vi "InternalGenerateValObjXML.vi"(6 "static class name":string, 7 "Class version":T1, 10 "Parent After Child":string, 11 "Parent Before Child":string) -> (0 "After Child":string, 1 "Object as XML":string, 3 "Before Child":string)   [LabVIEW 2015, in "OpenG_Value_Object.lvclass"]
doc: "A method used internally by the class to construct XML."
uses:
  <userlib>/_OpenG.lib/openg_object/openg_value_object.llb/OpenG_Value_Object.lvclass
  <userlib>/_OpenG.lib/openg_object/openg_object.llb/OpenG_Object.lvclass
panel:
  # "Please visit http://www.OpenG.org to learn about the\nOpen Source LabVIEW software movement.\n\nNOTICE -- YOU MUST LEAVE THIS NOTICE IN PLACE.  PER THE TERMS OF THE LICENSE BELOW, YOU MAY SUBLICENSE THIS SOFTWARE \nIN ANY WAY THAT DOES NOT CONFLICT WITH THIS LICENSE.\n\n### BSD License (http://www.opensource.org/licenses/bsd-license.php) Begin ###\n\nCopyright (c) 2007, Tomi Maila\nCopyright (c) 2007, Endevo AB\n\n\nAll rights reserved.\n\nRedistribution and use in source and binary forms, with or without modification, are permitted provided that the following conditions are met:\n\n    * Redistributions of source code must retain the above copyright notice, this list of conditions and the following disclaimer.\n    * Redistributions in binary form must reproduce the above copyright notice, this list of conditions and the following disclaimer in the \n       documentation and/or other materials provided with the distribution.\n    * Neither the name of Endevo AB nor the names of the contributors may be used to endorse or promote products derived\n       from this software without specific prior written permission.\n\nTHIS SOFTWARE IS PROVIDED BY THE COPYRIGHT HOLDERS AND CONTRIBUTORS \"AS IS\" AND ANY EXPRESS OR IMPLIED WARRANTIES, \nINCLUDING, BUT NOT LIMITED TO, THE IMPLIED WARRANTIES OF MERCHANTABILITY AND FITNESS FOR A PARTICULAR PURPOSE ARE \nDISCLAIMED. IN NO EVENT SHALL THE COPYRIGHT OWNER OR CONTRIBUTORS BE LIABLE FOR ANY DIRECT, INDIRECT, INCIDENTAL,\n SPECIAL, EXEMPLARY, OR CONSEQUENTIAL DAMAGES (INCLUDING, BUT NOT LIMITED TO, PROCUREMENT OF SUBSTITUTE GOODS OR \nSERVICES; LOSS OF USE, DATA, OR PROFITS; OR BUSINESS INTERRUPTION) HOWEVER CAUSED AND ON ANY THEORY OF LIABILITY, \nWHETHER IN CONTRACT, STRICT LIABILITY, OR TORT (INCLUDING NEGLIGENCE OR OTHERWISE) ARISING IN ANY WAY OUT OF THE USE \nOF THIS SOFTWARE, EVEN IF ADVISED OF THE POSSIBILITY OF SUCH DAMAGE.\n\n### BSD License End ###"
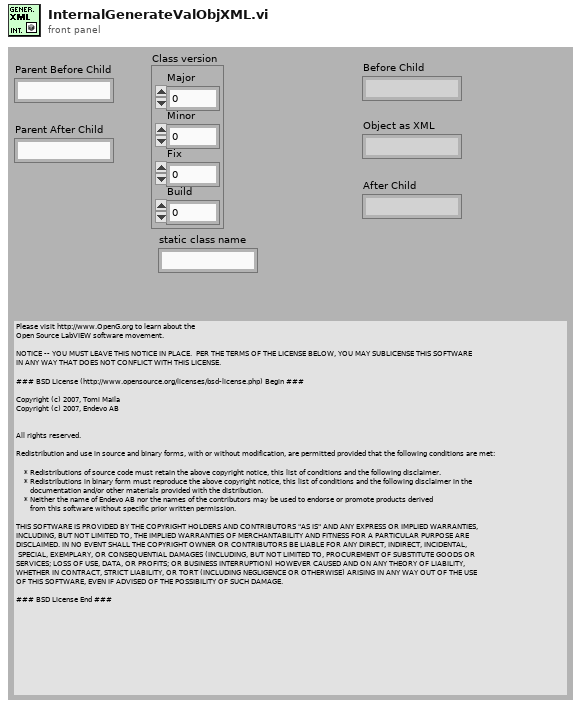
[diagram p1: front panel]
types:
  T1 = cluster{"Major":u16, "Minor":u16, "Fix":u16, "Build":u16}
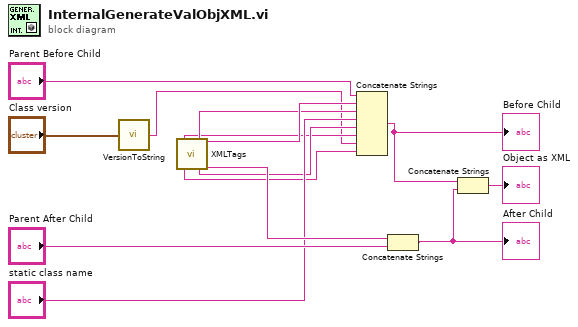
[diagram p0: block diagram]
diagram:
  n1 = call <userlib>:"VersionToString.vi"("Version"="Class version") -> ("Version as string"=w2:string)
  n2 = call <userlib>:"XMLTags.vi"() -> ("<Version>"=w3:string, "</Version>"=w1:string, "<Type>"=w6:string, "</Type>"=w4:string, "<Class>"=w8:string, "</Class>"=w12:string)  [unwired: 4 in, 10 out]
  n3 = Concatenate Strings("Parent Before Child", w8, w6, "static class name", w4, w3, w2, w1) -> (w11:string)
  "Before Child" <- w11
  n4 = Concatenate Strings(w12, "Parent After Child") -> (w13:string)
  "After Child" <- w13
  n5 = Concatenate Strings(w11, w13) -> (→"Object as XML":string)
